vi "TLMotorStopCtrl.vi"(4 "Error In (No Error)":errorcluster, 7 "Motor Ref":refnum<k7>) -> (0 "Error Out":errorcluster, 3 "Motor Ref":refnum<k7>)   [LabVIEW 2014]
doc: "Stops the Motor control.\n\nIn\nMotor Ref - Reference to Motor control object.\nError In (No Error) - Standard LabView error cluster.\n\nOut\nMotor Ref - Reference to Motor control object.\nError Out - Standard LabView error cluster."
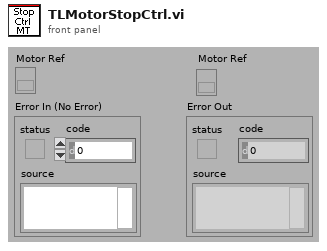
[diagram p1: front panel]
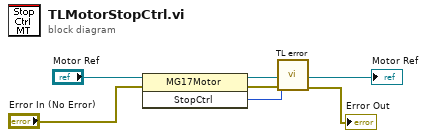
[diagram p0: block diagram]
diagram:
  n1 = invoke class="MG17Motor" method="StopCtrl"(reference="Motor Ref", error in="Error In (No Error)") -> (reference out=→"Motor Ref":refnum<k7>, error out=w5:errorcluster, "StopCtrl"=w3:i32)  [unwired: 1 in]
  n2 = call "TL error.vi"("error in (no error)"=w5, "Return Code"=w3) -> ("error out"=→"Error Out":errorcluster)  [unwired: 9 in]
